vi "IPI_ROI_Set.vi"(8 "元素":i32, 9 "Y":i32=5, 10 "X":i32, 11 "XYCenter":cluster{"X":i32, "Y":i32}) -> (3 "ROI":T1)   [LabVIEW 2015]
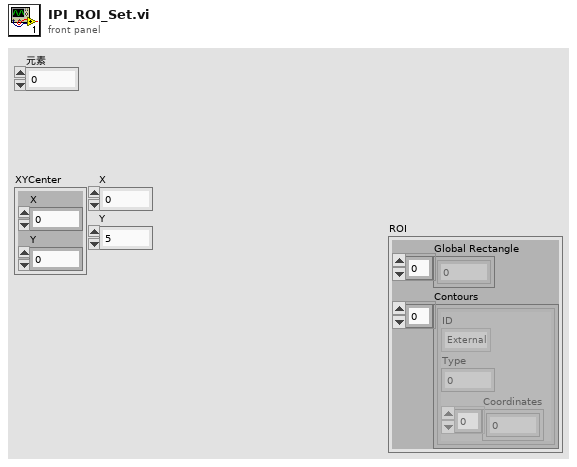
[diagram p1: front panel]
types:
  T1 = cluster{"Global Rectangle":i32[], "Contours":cluster{"ID":enum32{"External", "Internal"}, "Type":u32, "Coordinates":i32[]}[]}
  T2 = cluster{"ID":enum32{"External", "Internal"}, "Type":u32, "Coordinates":i32[]}
  T3 = cluster{"ID":enum32{"External", "Internal"}, "Type":u32, "Coordinates":i32[]}[]
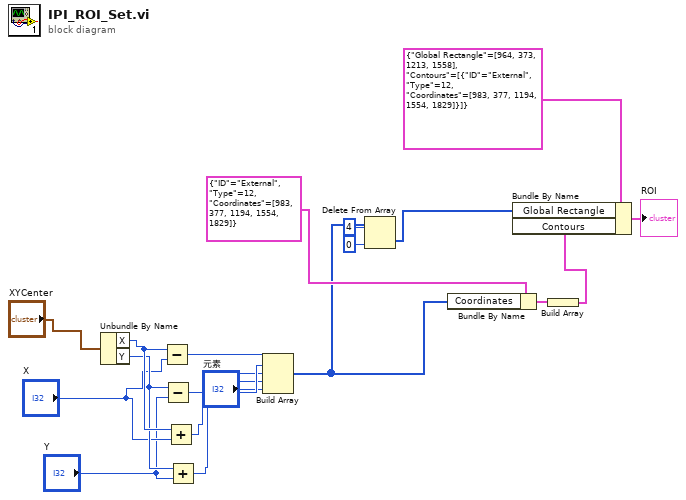
[diagram p0: block diagram]
diagram:
  n1 = Unbundle By Name("XYCenter") -> ("X"=w13:i32, "Y"=w12:i32)
  n2 = Subtract(x=w13, y="X") -> (x-y=w11:i32)
  n3 = Subtract(x=w12, y="Y") -> (x-y=w10:i32)
  n4 = Add(x=w13, y="X") -> (x+y=w9:i32)
  n5 = Add(x=w12, y="Y") -> (x+y=w8:i32)
  n6 = Build Array(w11, w10, w9, w8, "元素") -> (w4:i32[])
  n7 = Delete From Array(array=w4, length=4 ("长度"), index=0 ("索引")) -> (deleted portion=w1:i32[])  [unwired: 1 out]
  n8 = Bundle By Name(cluster=T2 {"ID"=enum."External", "Type"=12, "Coordinates"=[983, 377, 1194, 1554, 1829]}, "Coordinates"=w4) -> (w18:T2)
  n9 = Build Array(w18) -> (w17:T3)
  n10 = Bundle By Name(cluster=T1 {"Global Rectangle"=[964, 373, 1213, 1558], "Contours"=[{"ID"=enum."External", "Type"=12, "Coordinates"=[983, 377, 1194, 1554, 1829]}]} ("ROI Descriptor (Find Straight Edge 1)"), "Global Rectangle"=w1, "Contours"=w17) -> (→"ROI":T1)
